vi "visionTrackingSubsystem Controller.vi"(8 "error in":errorcluster) -> ()   [LabVIEW 2015]
doc: "This VI executes continuously carrying out the current operation and responding to updates or new operations. It will often contain the timing or control code that is difficult to place directly in TeleOp. This VI generally opens all sensors and motors and isolates the rest of the robot code from knowing how the operations are carried out."
uses:
  visionTrackingSubsystem Setpoints.ctl
  visionTrackingSubsystem Operations.ctl
  <vilib>/Rock Robotics/WPI/Camera/WPI_CameraImageSize.ctl
  <vilib>/Rock Robotics/WPI/MotorControl/WPI_MotorControlOpenCANTalonSRX.vi
  <vilib>/addons/control/pid/pid.llb/PID (DBL).vi
  <vilib>/Rock Robotics/Network Tables/NT Write Boolean.vi
  <vilib>/addons/control/pid/NI_PID_pid.lvlib
panel:
  in  "D":dbl
  in  "I":dbl
  in  "P":dbl
  out "Current\nCmd":string
  # "Tip: It may be helpful to observe inputs and sensor values.\nYou may also want to display tuning or debugging controls."
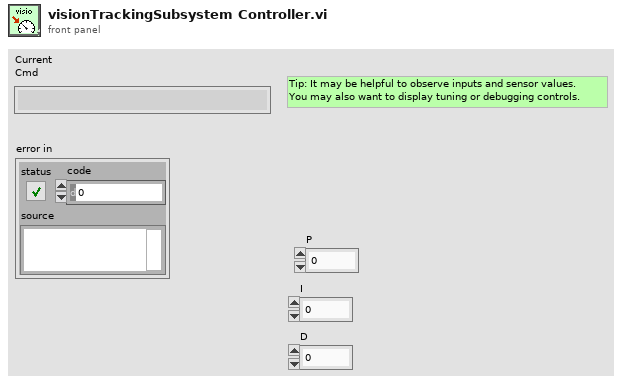
[diagram p1: front panel]
types:
  T1 = typedef "visionTrackingSubsystem Setpoints.ctl" = cluster{"Operation":T2, "Setpoint":dbl, "Duration":dbl}
  T2 = typedef "visionTrackingSubsystem Operations.ctl" = enum16{"Reserve", "Read Current", "Immediate"}
  T3 = typedef "WPI_MotorControlDeviceRef.ctl" = cluster{"DeviceStatus":errorcluster, "Type":T4, "PWM":cluster{"PWM Channel":T5, "DeadBand":T6}, "CAN":cluster{"Device Number":u8, "Control Mode":T7, "Semaphore":T8, "Max Vout":dbl, "TalonSRX Control Mode":T9}, "Invert":bool}
  T4 = typedef "WPI_MotorControlType.ctl" = enum16{"PWM", "CAN", "CANTalonSRX"}
  T5 = typedef "FPGA_DIOPWMChannel.ctl" = enum8{"PWM 0", "PWM 1", "PWM 2", "PWM 3", "PWM 4", "PWM 5", "PWM 6", "PWM 7", "PWM 8", "PWM 9", "PWM MXP 0", "PWM MXP 1", "PWM MXP 2", "PWM MXP 3", "PWM MXP 4", "PWM MXP 5", "PWM MXP 6", "PWM MXP 7", "PWM MXP 8", "PWM MXP 9", "Invalid"}
  T6 = typedef "WPI_PWMDeadband.ctl" = cluster{"Name":string, "maxPositivePwm":i32, "minPositivePwm":i32, "centerPwm":i32, "maxNegativePwm":i32, "minNegativePwm":i32, "angularRange":u16}
  T7 = typedef "WPI_CANJaguar_ControlMode.ctl" = enum8{"Percent VBus", "Current", "Speed", "Position", "Voltage"}
  T8 = typedef "Semaphore RefNum" = refnum<k1>
  T9 = typedef "WPI_CANTalonSRX_APIControlMode.ctl" = enum8{"Percent VBus", "Speed", "Position", "Slave", "Unchanged / Invalid", "Voltage Compensation", "Current", "Motion Profile"}
  T10 = typedef "Command Status Info.ctl" = cluster{"Name":string, "Status":T11, "notifier out":T12}
  T11 = typedef "Completion Status.ctl" = enum16{"Successful", "Aborted", "Incomplete"}
  T12 = typedef "Completion Notifier.ctl" = refnum<notifier>
  T13 = cluster{"Default Command":T1, "Command Timing":cluster{"Start Time (ms)":u32, "Iterations":i32}, "Command Arguments":cluster{"Command Info":T10, "Description":string, "Default Command":T1, "notifier out":refnum<notifier>, "Subsystem Name":string}}
  T14 = typedef "WPI_CameraImageSize.ctl" = enum16{"640x480", "320x240", "160x120", "Custom"}
  T15 = cluster{"Distance (ft)":dbl, "Center":cluster{dbl, dbl}, "Normalized Rect":cluster{"Numeric":dbl, "Numeric 2":dbl, "Numeric 3":dbl, "Numeric 5":dbl}}[]
  T16 = cluster{"Distance (ft)":dbl, "Center":cluster{dbl, dbl}, "Normalized Rect":cluster{"Numeric":dbl, "Numeric 2":dbl, "Numeric 3":dbl, "Numeric 5":dbl}}
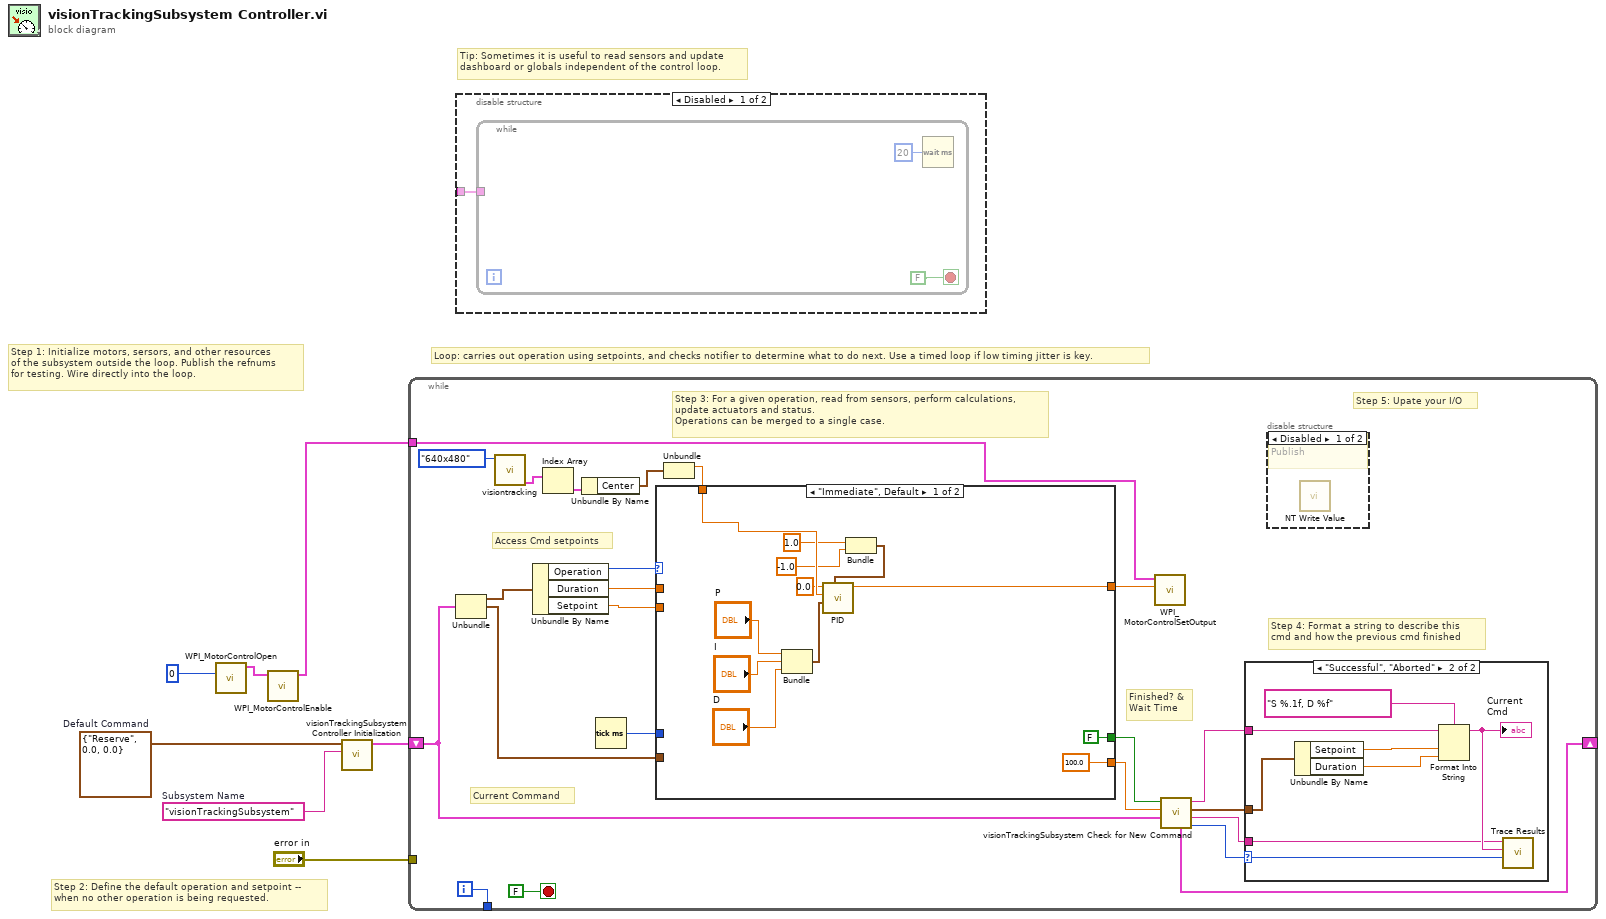
[diagram p0: block diagram]
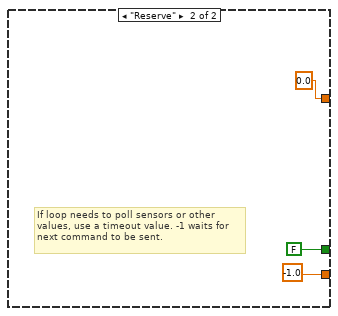
[diagram p5: hidden frame]
diagram:
  w4 = T1 {"Operation"=enum."Reserve", "Setpoint"=0.0, "Duration"=0.0}  # Default Command
  w5 = "visionTrackingSubsystem"  # Subsystem Name
  # "Tip: Sometimes it is useful to read sensors and update\ndashboard or globals independent of the control loop."
  # "Step 2: Define the default operation and setpoint --\nwhen no other operation is being requested."
  # "Step 1: Initialize motors, sersors, and other resources\nof the subsystem outside the loop. Publish the refnums\nfor testing. Wire directly into the loop."
  # "Loop: carries out operation using setpoints, and checks notifier to determine what to do next. Use a timed loop if low timing jitter is key."
  n1 = call-poly <vilib>:"WPI_MotorControlOpen.vi"("Device Number"=u8 0) -> ("MotorControlDeviceRef"=w3:T3)  [unwired: 9 in, 1 out]
  n2 = call <vilib>:"WPI_MotorControlEnable.vi"("CAN MotorDevRef"=w3) -> ("CAN MotorDevRef"=w1:T3)  [unwired: 9 in, 1 out]
  n3 = call "visionTrackingSubsystem Controller Initialization.vi"("Subsystem Name"=w5, "Default Command"=w4) -> ("Command Info"=w6:T13)  [unwired: 9 in]
  n4 = while {
    shift-right: [w21] -> _
    shift-left: w6 -> [w22]
    tunnel: [w29] -> _
    tunnel: "error in" -> [_]
    tunnel: w1 -> [w9]
    i -> [w29]
    stop <- FALSE stop-if-true
    # "Step 5: Upate your I/O"
    # "Step 4: Format a string to describe this\ncmd and how the previous cmd finished"
    # "Current Command"
    # "Access Cmd setpoints"
    # "Finished? &\nWait Time"
    # "Step 3: For a given operation, read from sensors, perform calculations,\nupdate actuators and status.\nOperations can be merged to a single case."
    n5 = Unbundle(w22) -> ("Default Command"=w28:T1, "Command Timing"=w24:cluster{"Start Time (ms)":u32, "Iterations":i32})  [unwired: 1 out]
    n6 = call "visiontracking.vi"("Image Size"=WPI_CameraImageSize."640x480") -> ("Detected Targets"=w13:T15)  [unwired: 6 in]
    n7 = Unbundle By Name(w28) -> ("Operation"=w27:T2, "Duration"=w26:dbl, "Setpoint"=w23:dbl)
    n8 = Index Array(array=w13) -> (element=w14:T16)  [unwired: 1 in]
    n9 = Unbundle By Name(w14) -> ("Center"=w11:cluster{dbl, dbl})
    n10 = Tick Count (ms)() -> (millisecond timer value=w25:u32)
    n11 = Unbundle(w11) -> (w8:dbl)  [unwired: 1 out]
    n12 = case shown="\"Immediate\", Default" w27 {
      tunnel: [100.0 -1.0] -> w19
      tunnel: [FALSE ("ignore previous (F)") FALSE ("ignore previous (F)")] -> w20
      tunnel: w24 -> [_ _]
      tunnel: w26 -> [_ _]
      tunnel: w25 -> [_ _]
      tunnel: w23 -> [_ _]
      tunnel: w8 -> [w49 _]
      tunnel: [w39 0.0 ("output")] -> w10
      frame "Immediate", Default {
        n13 = Bundle("P"="P", "I"="I", "D"="D") -> (w44:cluster{"P":dbl, "I":dbl, "D":dbl})  [unwired: 1 in]
        n14 = Bundle(1.0, -1.0) -> (w41:cluster{dbl, dbl})  [unwired: 1 in]
        n15 = call-poly <vilib>:"PID.vi"("output range"=w41, "PID gains"=w44, "process variable"=w49, "setpoint"=0.0) -> ("output"=w39:dbl)  [unwired: 6 in, 1 out]
      }
      frame "Reserve" {
        # "If loop needs to poll sensors or other\nvalues, use a timeout value. -1 waits for\nnext command to be sent."
      }
    }
    n16 = call <vilib>:"WPI_MotorControlSetOutput.vi"("Output"=w10, "MotorControlDevRef"=w9) -> ()  [unwired: 7 in, 3 out]
    n17 = call "visionTrackingSubsystem Check for New Command.vi"("Current Command"=w22, "Wait time (ms)"=w19, "Finished?"=w20) -> ("Completion"=w15:T11, "Subsystem Name"=w16:string, "Current Command"=w17:T1, "Initial Trace String"=w18:string, "NextCommand"=w21:T13)  [unwired: 4 in]
    n18 = case shown="\"Successful\", \"Aborted\"" w15 {
      selector: w15 -> [_ w38]
      tunnel: w18 -> [_ w34]
      tunnel: w17 -> [_ w35]
      tunnel: w16 -> [_ w31]
      frame "Incomplete", Default {
        # "Continuing current command"
      }
      frame "Successful", "Aborted" {
        # "Report and setup for next command"
        n19 = Unbundle By Name(w35) -> ("Setpoint"=w37:dbl, "Duration"=w32:dbl)
        n20 = Format Into String(format string="S %.1f, D %f", initial string=w34, w37, w32) -> (resulting string=w33:string)  [unwired: 1 in, 1 out]
        "Current\nCmd" <- w33
        n21 = call <vilib>:"Trace Results.vi"("Status of previous command"=w38, "Description"=w33, "Subsystem"=w31) -> ()  [unwired: 9 in]
      }
    }
    n22 = disable-structure shown="Disabled" {
      frame Disabled {
        # "Publish"
        n23 = call-poly <vilib>:"NT Write Value.vi"() -> ()  [unwired: 11 in, 1 out]
      }
      frame Enabled {
      }
    }
  }
  n24 = disable-structure shown="Disabled" {
    disable-tunnel: _ -> [w54 _]
    frame Disabled {
      n25 = while {
        tunnel: w54 -> [_]
        stop <- FALSE stop-if-true
        n26 = Wait (ms)(milliseconds to wait=u32 20) -> ()  [unwired: 1 out]
      }
    }
    frame Enabled {
    }
  }
